vi "takeCube.vi"(5 "ChangeCubes":bool, 7 "LeftArm":bool, 8 "Error/Flow In":errorcluster, 9 "Position (mm)":cluster{"X":dbl, "Y":dbl, "Theta":dbl}, 10 "theta":dbl) -> (0 "error out":errorcluster, 1 "Position Out":cluster{"X":dbl, "Y":dbl, "Theta":dbl})   [LabVIEW 2018]
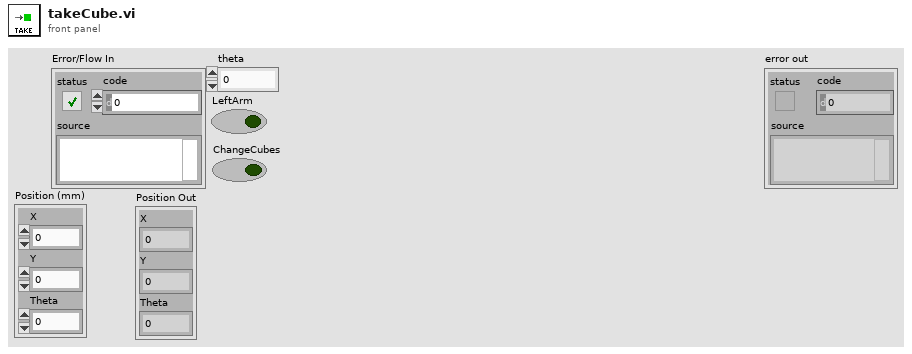
[diagram p1: front panel]
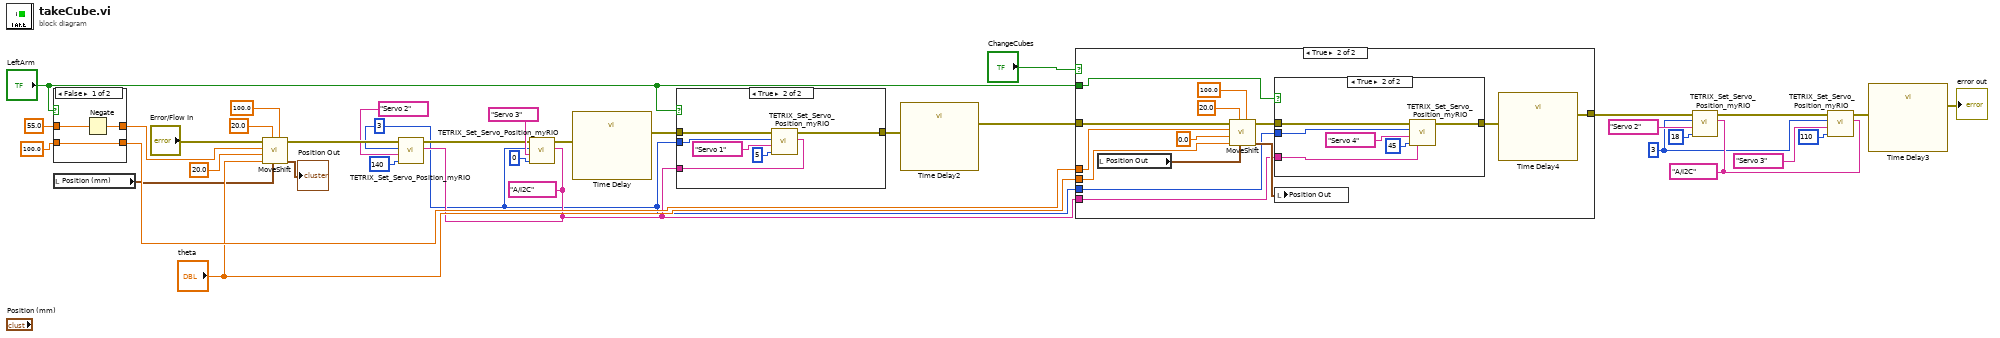
[diagram p0: block diagram]
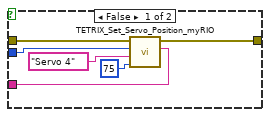
[diagram p2: hidden frame]
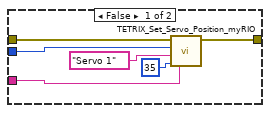
[diagram p4: hidden frame]
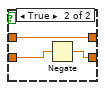
[diagram p5: hidden frame]
diagram:
  w5 = u8 3 ("Controller ID#  (I2C Address)")
  w7 = tag "A/I2C" ("myRIO MXP Port A/B")
  w13 = u8 3 ("Controller ID#  (I2C Address)")
  w14 = tag "A/I2C" ("myRIO MXP Port A/B")
  n1 = case shown="False" "LeftArm" {
    tunnel: 55.0 ("x shift") -> [w38 w41]
    tunnel: [w37 w41] -> w30
    tunnel: 100.0 ("x shift") -> [w36 w40]
    tunnel: [w36 w39] -> w17
    frame False {
      n2 = Negate(x=w38) -> (-x=w37:dbl)
    }
    frame True {
      n3 = Negate(x=w40) -> (-x=w39:dbl)
    }
  }
  n4 = local read "Position (mm)"() -> (w1:cluster{"X":dbl, "Y":dbl, "Theta":dbl})
  n5 = call "MoveShift.vi"("max speed"=100.0, "Position"=w1, "Precision"=20.0, "theta"="theta", "y shift"=20.0, "x shift"=w30, "Error/Flow In"="Error/Flow In") -> ("Position Out"=→"Position Out":cluster{"X":dbl, "Y":dbl, "Theta":dbl}, "Error/Flow Out"=w29:errorcluster)  [unwired: 3 in]
  n6 = call <vilib>:"TETRIX_Set_Servo_Position_myRIO.vi"("myRIO MXP Port A/B"=w14, "Set Servo Position (0 - 180 degrees)"=u8 140, "Select Channel"="Servo 2", "Controller ID#  (I2C Address)"=w13, "Error/Flow In"=w29) -> ("Error/Flow Out"=w24:errorcluster)  [unwired: 2 in]
  n7 = call <vilib>:"TETRIX_Set_Servo_Position_myRIO.vi"("myRIO MXP Port A/B"=w14, "Set Servo Position (0 - 180 degrees)"=u8 0, "Select Channel"="Servo 3", "Controller ID#  (I2C Address)"=w13, "Error/Flow In"=w24) -> ("Error/Flow Out"=w23:errorcluster)  [unwired: 2 in]
  n8 = call "Time Delay"("error in (no error)"=w23) -> ("error out"=w22:errorcluster)  [unwired: 10 in]
  n9 = case shown="True" "LeftArm" {
    tunnel: w22 -> [w45 w53]
    tunnel: w14 -> [w44 w52]
    tunnel: w13 -> [w43 w51]
    tunnel: [w42 w48] -> w21
    frame False {
      n10 = call <vilib>:"TETRIX_Set_Servo_Position_myRIO.vi"("myRIO MXP Port A/B"=w44, "Set Servo Position (0 - 180 degrees)"=u8 75, "Select Channel"="Servo 4", "Controller ID#  (I2C Address)"=w43, "Error/Flow In"=w45) -> ("Error/Flow Out"=w42:errorcluster)  [unwired: 2 in]
    }
    frame True {
      n11 = call <vilib>:"TETRIX_Set_Servo_Position_myRIO.vi"("myRIO MXP Port A/B"=w52, "Set Servo Position (0 - 180 degrees)"=u8 5, "Select Channel"="Servo 1", "Controller ID#  (I2C Address)"=w51, "Error/Flow In"=w53) -> ("Error/Flow Out"=w48:errorcluster)  [unwired: 2 in]
    }
  }
  n12 = call "Time Delay2"("error in (no error)"=w21) -> ("error out"=w19:errorcluster)  [unwired: 10 in]
  n13 = case shown="True" "ChangeCubes" {
    tunnel: w19 -> [w54 w63]
    tunnel: w17 -> [_ w66]
    tunnel: "theta" -> [_ w64]
    tunnel: "LeftArm" -> [_ w60]
    tunnel: w14 -> [_ w58]
    tunnel: w13 -> [_ w57]
    tunnel: [w54 w55] -> w6
    frame False {
    }
    frame True {
      n14 = local read "Position Out"() -> (w68:cluster{"X":dbl, "Y":dbl, "Theta":dbl})
      n15 = call "MoveShift.vi"("max speed"=100.0, "Position"=w68, "Precision"=20.0, "theta"=w64, "y shift"=0.0, "x shift"=w66, "Error/Flow In"=w63) -> ("Position Out"=w67:cluster{"X":dbl, "Y":dbl, "Theta":dbl}, "Error/Flow Out"=w59:errorcluster)  [unwired: 3 in]
      n16 = case shown="True" w60 {
        tunnel: w59 -> [w72 w78]
        tunnel: w58 -> [w71 w77]
        tunnel: w57 -> [w70 w76]
        tunnel: [w69 w75] -> w56
        frame False {
          n17 = call <vilib>:"TETRIX_Set_Servo_Position_myRIO.vi"("myRIO MXP Port A/B"=w71, "Set Servo Position (0 - 180 degrees)"=u8 35, "Select Channel"="Servo 1", "Controller ID#  (I2C Address)"=w70, "Error/Flow In"=w72) -> ("Error/Flow Out"=w69:errorcluster)  [unwired: 2 in]
        }
        frame True {
          n18 = call <vilib>:"TETRIX_Set_Servo_Position_myRIO.vi"("myRIO MXP Port A/B"=w77, "Set Servo Position (0 - 180 degrees)"=u8 45, "Select Channel"="Servo 4", "Controller ID#  (I2C Address)"=w76, "Error/Flow In"=w78) -> ("Error/Flow Out"=w75:errorcluster)  [unwired: 2 in]
        }
      }
      n19 = local write "Position Out"(w67) -> ()
      n20 = call "Time Delay4"("error in (no error)"=w56) -> ("error out"=w55:errorcluster)  [unwired: 10 in]
    }
  }
  n21 = call <vilib>:"TETRIX_Set_Servo_Position_myRIO.vi"("myRIO MXP Port A/B"=w7, "Set Servo Position (0 - 180 degrees)"=u8 18, "Select Channel"="Servo 2", "Controller ID#  (I2C Address)"=w5, "Error/Flow In"=w6) -> ("Error/Flow Out"=w8:errorcluster)  [unwired: 2 in]
  n22 = call <vilib>:"TETRIX_Set_Servo_Position_myRIO.vi"("myRIO MXP Port A/B"=w7, "Set Servo Position (0 - 180 degrees)"=u8 110, "Select Channel"="Servo 3", "Controller ID#  (I2C Address)"=w5, "Error/Flow In"=w8) -> ("Error/Flow Out"=w4:errorcluster)  [unwired: 2 in]
  n23 = call "Time Delay3"("error in (no error)"=w4) -> ("error out"=→"error out":errorcluster)  [unwired: 10 in]
